vi "Instrument Status Register.vi"(8 "error in (no error)":errorcluster, 11 "VISA resource name":refnum<visa-resource-name>) -> (0 "error out":errorcluster, 1 "Instrument Status Register Values":T1, 2 "Instrument Status Register":i32, 3 "VISA resource name out":refnum<visa-resource-name>, 4 "Device Errors":cluster{"code":i32, "Text":string}[](array[cluster]))   [LabVIEW 2014, in "Stanford Research DG645 - Driver.lvlib"]
doc: "Status and Display Command: INSR?\nInstrument Error Check\n\nQuery the Instrument Status Register. Upon Executing a INSR? query, the returned bits of the INSR register are cleared. The bits in the INSR register have the following meaning:\n\nBit Meaning\n0 Got a trigger\n1 Got a trigger while a delay or burst\n was in progress\n2 a delay cycle has completed\n3 a burst cycle has completed\n4 a trigger or output delay cycle was\n inhibited\n5 a delay cycle was aborted early\n6 the 100MHz PLL came unlocked\n7 the installed Rb oscillator is unlocked"
uses:
  Stanford Research DG645 - Driver.lvlib
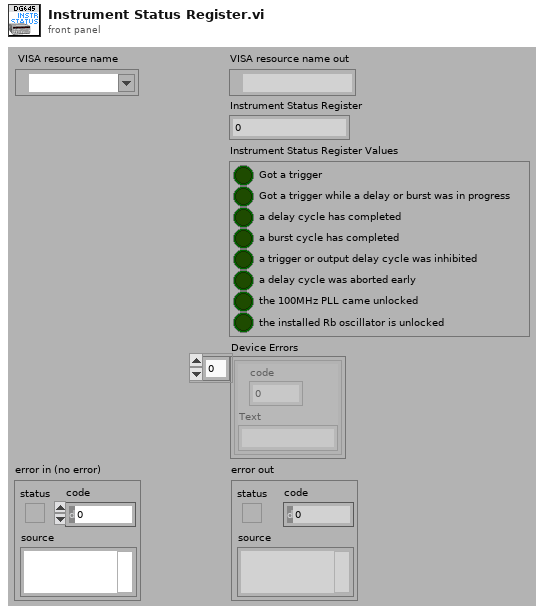
[diagram p1: front panel]
types:
  T1 = cluster{"Got a trigger":bool, "Got a trigger while a delay or burst was in progress":bool, "a delay cycle has completed":bool, "a burst cycle has completed":bool, "a trigger or output delay cycle was inhibited":bool, "a delay cycle was aborted early":bool, "the 100MHz PLL came unlocked":bool, "the installed Rb oscillator is unlocked":bool}
  T2 = cluster{"Boolean array[0]":bool, "Boolean array[1]":bool, "Boolean array[2]":bool, "Boolean array[3]":bool, "Boolean array[4]":bool, "Boolean array[5]":bool, "Boolean array[6]":bool, "Boolean array[7]":bool}
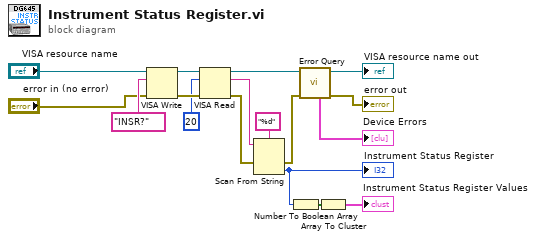
[diagram p0: block diagram]
diagram:
  n1 = VISA Write(VISA resource name="VISA resource name", write buffer="INSR?" ("Self-Test Command"), error in (no error)="error in (no error)") -> (VISA resource name out=w16:refnum<visa-resource-name>, error out=w15:errorcluster)  [unwired: 1 out]
  n2 = VISA Read(VISA resource name=w16, byte count=u32 20 ("byte count (20)"), error in (no error)=w15) -> (VISA resource name out=w5:refnum<visa-resource-name>, read buffer=w13:string, error out=w8:errorcluster)  [unwired: 1 out]
  n3 = Scan From String(format string="%d", input string=w13, error in=w8) -> (error out=w4:errorcluster, output 1=w3:i32)  [unwired: 2 in, 2 out]
  "Instrument Status Register" <- w3
  n4 = Number To Boolean Array(number=w3) -> (Boolean array=w2:bool[])
  n5 = call "Error Query.vi"("error in (no error)"=w4, "VISA resource name"=w5) -> ("error out"=→"error out":errorcluster, "VISA resource name out"=→"VISA resource name out":refnum<visa-resource-name>, "Device Errors"=→"Device Errors":cluster{"code":i32, "Text":string}[])  [unwired: 7 in]
  n6 = Array To Cluster(array=w2) -> (cluster=→"Instrument Status Register Values":T2)
